vi "GenNet Version-Safe Unflatten Variant.vi"(8 "error in":errorcluster, 11 "Flattened Data":string) -> (0 "error out":errorcluster, 3 "Message Data":variant)   [LabVIEW 2020, in "hse-gennet.lvlib"]
doc: "Unflattens a variant from a string. Automatically prepends the correct header if the variant was flattened in another LabVIEW version.\n\n____\nHAMPEL SOFTWARE ENGINEERING v3.8.0 (2023-12-18 14:41)"
uses:
  hse-gennet.lvlib
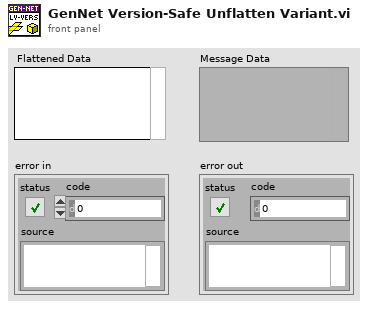
[diagram p1: front panel]
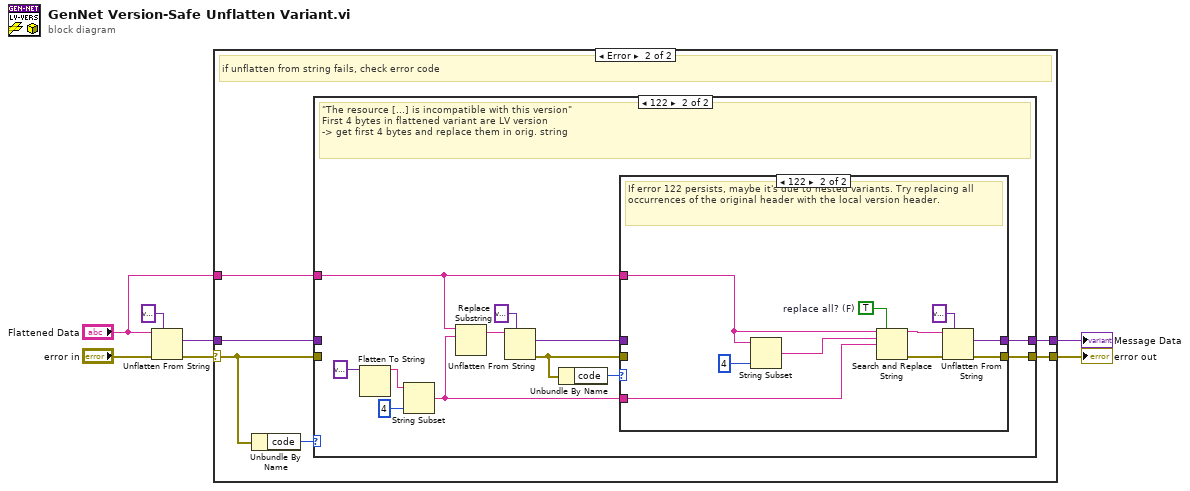
[diagram p0: block diagram]
diagram:
  n1 = Unflatten From String(type=variant ("Message Data"), binary string="Flattened Data", error in (no error)="error in") -> (value=w6:variant, error out=w4:errorcluster)  [unwired: 2 in, 1 out]
  n2 = case shown="Error" w4 {
    selector: w4 -> [w9 w14]
    tunnel: w6 -> [w8 w12]
    tunnel: [w9 w13] -> w3
    tunnel: [w8 w11] -> w2
    tunnel: "Flattened Data" -> [_ w10]
    frame No Error {
    }
    frame Error {
      # "if unflatten from string fails, check error code"
      n3 = Unbundle By Name(w14) -> ("code"=w15:i32)
      n4 = case shown="122" w15 {
        tunnel: w14 -> [w17 _]
        tunnel: [w17 w20] -> w13
        tunnel: w12 -> [w16 _]
        tunnel: [w16 w22] -> w11
        tunnel: w10 -> [_ w19]
        frame Default {
          # "Forward all errors"
        }
        frame 122 {
          # "\"The resource [...] is incompatible with this version\"\nFirst 4 bytes in flattened variant are LV version\n-> get first 4 bytes and replace them in orig. string"
          n5 = Flatten To String(anything=variant) -> (data string=w28:string)  [unwired: 3 in, 2 out]
          n6 = String Subset(string=w28, length (rest)=4 ("length (rest)")) -> (substring=w18:string)  [unwired: 1 in]
          n7 = Replace Substring(4:w18, 5:w19) -> (1:w25:string)  [unwired: 2 in, 1 out]
          n8 = Unflatten From String(type=variant ("Message Data"), binary string=w25) -> (value=w23:variant, error out=w21:errorcluster)  [unwired: 3 in, 1 out]
          n9 = Unbundle By Name(w21) -> ("code"=w24:i32)
          n10 = case shown="122" w24 {
            tunnel: w23 -> [w31 _]
            tunnel: [w31 w39] -> w22
            tunnel: w21 -> [w30 _]
            tunnel: [w30 w40] -> w20
            tunnel: w19 -> [_ w34]
            tunnel: w18 -> [_ w35]
            frame Default {
            }
            frame 122 {
              w36 = TRUE  # replace all? (F)
              # "If error 122 persists, maybe it's due to nested variants. Try replacing all occurrences of the original header with the local version header."
              n11 = String Subset(string=w34, length (rest)=4 ("length (rest)")) -> (substring=w32:string)  [unwired: 1 in]
              n12 = Search and Replace String(replace all?=w36, input string=w34, search string=w32, replace string=w35) -> (result string=w38:string, error out=w37:errorcluster)  [unwired: 4 in, 2 out]
              n13 = Unflatten From String(type=variant ("Message Data"), binary string=w38, error in (no error)=w37) -> (value=w39:variant, error out=w40:errorcluster)  [unwired: 2 in, 1 out]
            }
          }
        }
      }
    }
  }
  "Message Data" <- w2
  "error out" <- w3
